vi "openCamHigh.vi"(8 "error in (no error)":errorcluster, 10 "Camera Opened":bool, 11 "Boolean in":refnum<vi>) -> (0 "error out":errorcluster, 1 "Cam Handle":u32, 2 "Ydim":u32, 3 "Xdim":u32)   [LabVIEW 2015]
uses:
  Public/Documents/SItoolkit/LabVIEW/Examples2015_6_0_2_9/Fast Examples/Open-Close Hardware/CamHandle.vi
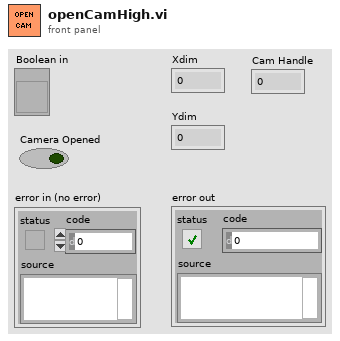
[diagram p1: front panel]
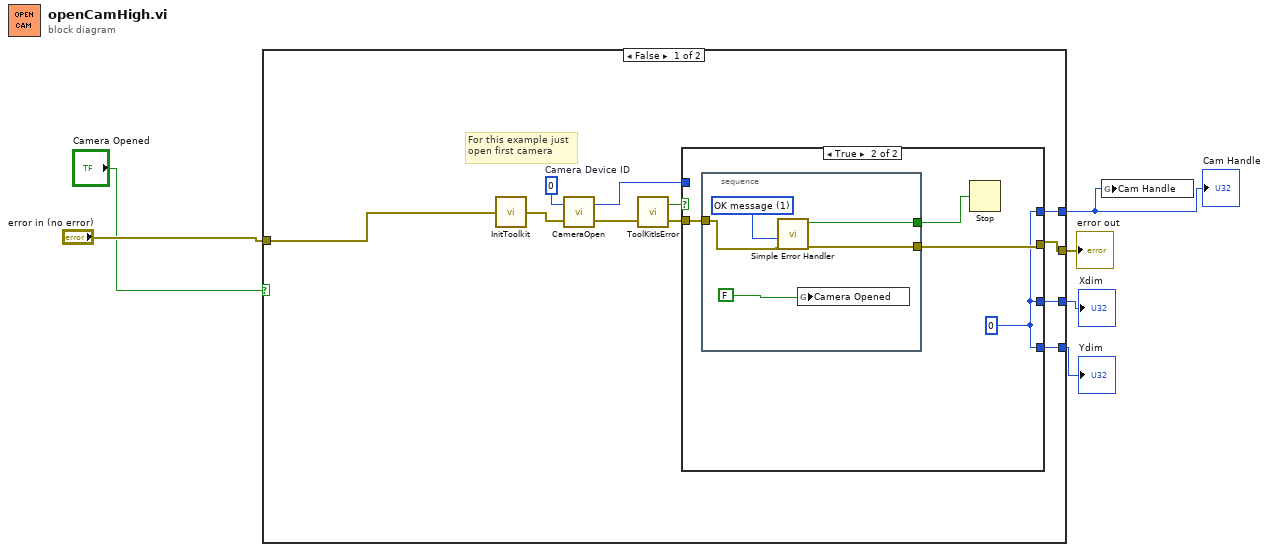
[diagram p0: block diagram]
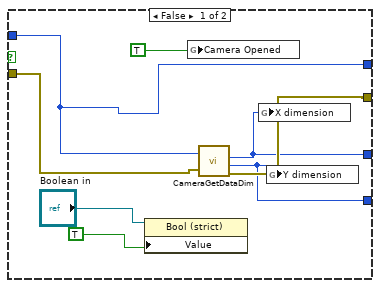
[diagram p2: hidden frame]
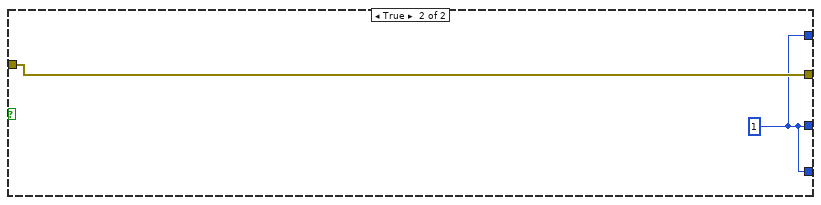
[diagram p3: hidden frame]
diagram:
  n1 = case shown="False" "Camera Opened" {
    tunnel: [w17 w35] -> w6
    tunnel: [w16 w35] -> w5
    tunnel: [w15 w36] -> w4
    tunnel: "error in (no error)" -> [w8 w36]
    tunnel: [w7 w35] -> w1
    frame False {
      w13 = u32 0  # Camera Device ID
      # "For this example just\nopen first camera"
      n2 = call <userlib>:"InitToolkit.vi"("error in"=w8) -> ("error out"=w9:errorcluster)
      n3 = call <userlib>:"CameraOpen.vi"("error in"=w9, "Camera Device ID"=w13) -> ("error out"=w10:errorcluster, "Camera Handle"=w14:u32)
      n4 = call <userlib>:"ToolKitIsError.vi"("error in"=w10) -> ("error out"=w12:errorcluster, "Error Flag"=w11:bool)  [unwired: 1 in]
      n5 = case shown="True" w11 {
        tunnel: w12 -> [w25 w29]
        tunnel: [w24 w28] -> w15
        tunnel: w14 -> [w18 _]
        tunnel: [w20 w26] -> w16
        tunnel: [w19 w26] -> w17
        tunnel: [w18 w26] -> w7
        frame False {
          n6 = property class="Bool (strict)"(reference="Boolean in", "Value"=TRUE) -> ()  [unwired: 1 in, 2 out]
          n7 = global write "CamHandle.vi" "Camera Opened"(TRUE) -> ()
          n8 = call <userlib>:"CameraGetDataDim.vi"("Camera Handle"=w18, "error in"=w25) -> ("Xdim"=w20:u32, "Ydim"=w19:u32, "error out"=w24:errorcluster)  [unwired: 1 out]
          n9 = global write "CamHandle.vi" "X dimension"(w20) -> ()
          n10 = global write "CamHandle.vi" "Y dimension"(w19) -> ()
        }
        frame True {
          w26 = 0
          n11 = stacked-sequence {
            tunnel: w29 -> [w33]
            tunnel: [w32] -> w27
            tunnel: [w31] -> w28
            frame #0 {
              w34 = u16 1 items=["no dialog", "OK message", "continue or stop message"] ("type of dialog (OK msg:1)")
              n12 = call <vilib>:"Simple Error Handler.vi"("type of dialog (OK msg:1)"=w34, "error in (no error)"=w33) -> ("error?"=w32:bool, "error out"=w31:errorcluster)  [unwired: 3 in, 3 out]
              n13 = global write "CamHandle.vi" "Camera Opened"(FALSE) -> ()
            }
          }
          n14 = Stop(stop? (T)=w27) -> ()
        }
      }
    }
    frame True {
      w35 = 1
    }
  }
  "Ydim" <- w6
  "Xdim" <- w5
  "error out" <- w4
  "Cam Handle" <- w1
  n15 = global write "CamHandle.vi" "Cam Handle"(w1) -> ()
